vi "Randomize.vi"(11 "Quantity":T1={"Name"="", "Value"=[], "Uncertainty"=[], "Degrees of Freedom"=[], "Correlation"=[], "Randomized uncertainty"=[]}) -> (1 "Canceled?":bool, 3 "Randomized Quantity":T1)   [LabVIEW 2013]
uses:
  qwtblvlib/TD Quantity.ctl
  <vilib>/gmath/statdist.llb/Normal Random.vi
  <vilib>/gmath/statdist.llb/Uniform Random.vi
  <vilib>/gmath/statdist.llb/Triangular Random.vi
  <vilib>/gmath/statdist.llb/Student t Random.vi
  <vilib>/gmath/NI_Gmath.lvlib
  <vilib>/Analysis/NI_AALBase.lvlib
  qwtblvlib/QWTBLVLib.lvlib
panel:
  in  "Repeats":i32=100 min=1 step=1
  out "no dof":bool
  out "msg":string
  in  "reload hist signal":bool
  out "Randomization for quantity:":string
  in  "Maximum - Mean":dbl=1.0 min=0.0
  in  "Mean - Minimum":dbl min=0.0
  in  "Distribution type":T2(ring)
  out "Degrees of freedom":i32=1 min=1
  out "Mean":dbl
  out "Uncertainty":dbl=1.0 min=1e-15
  in  "Seed":i32=-1
  in  "Cancel Button":bool
  in  "OK Button":bool
  out "Example histogram of 1000 samples":T3(graph)
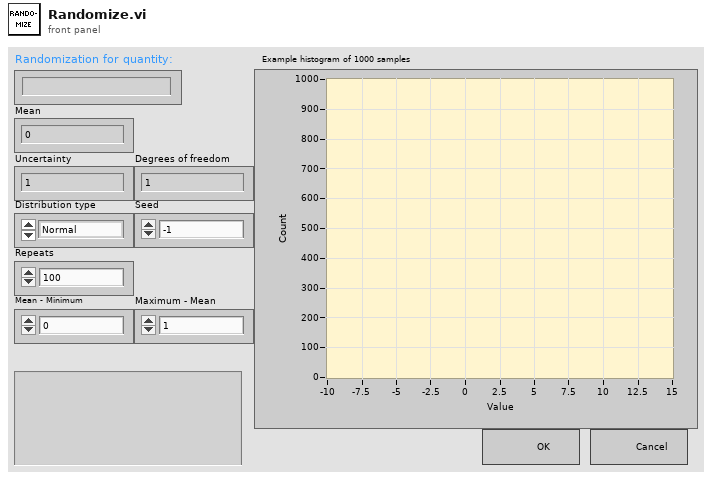
[diagram p1: front panel]
types:
  T1 = typedef "QWTBLVLib.lvlib/TD Quantity.ctl" = cluster{"Name":string, "Value":dbl[][], "Uncertainty":dbl[][], "Degrees of Freedom":dbl[][], "Correlation":dbl[][], "Randomized uncertainty":dbl[][]}
  T2 = enum16{"Normal", "t (Student)", "Triangular", "Uniform"}
  T3 = cluster{"X Values":dbl[], "Histogram: h(x)":i32[]}
  T4 = enum8{"Enabled", "Disabled", "Disabled and Grayed Out"}
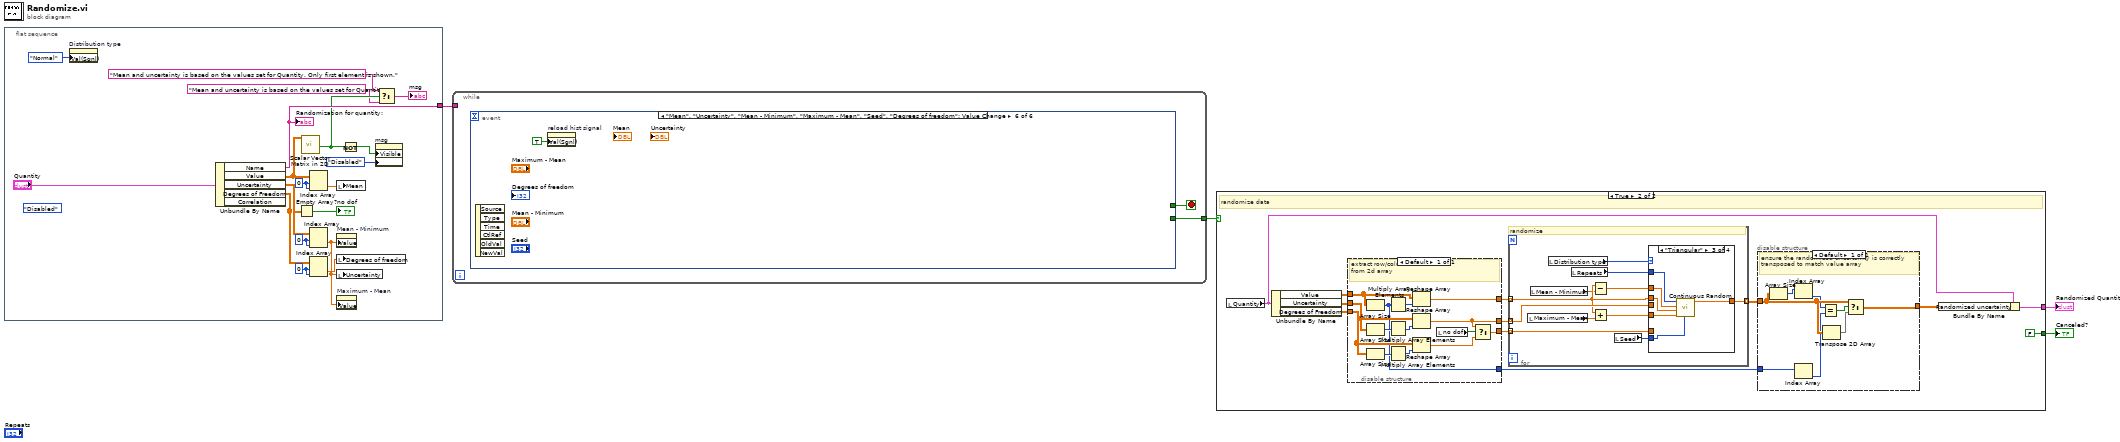
[diagram p0: block diagram]
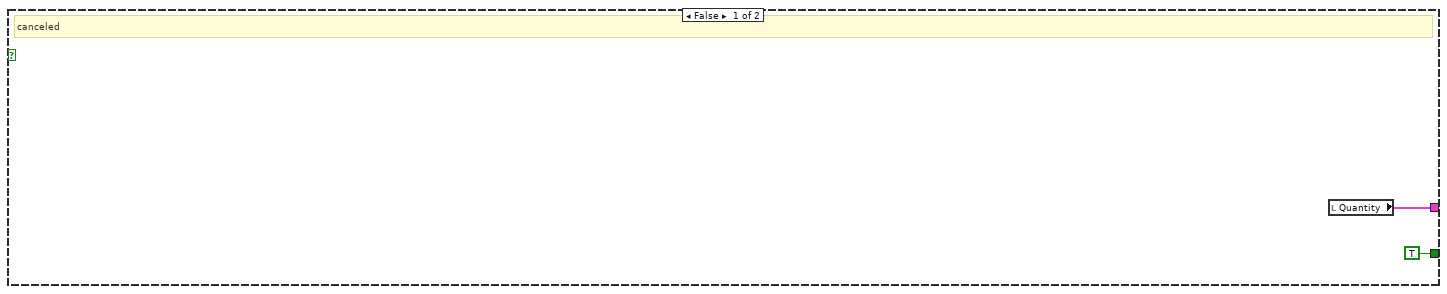
[diagram p2: hidden frame]
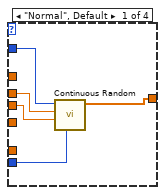
[diagram p3: hidden frame]
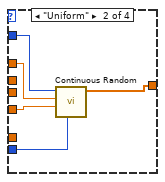
[diagram p4: hidden frame]
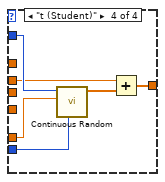
[diagram p5: hidden frame]
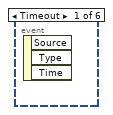
[diagram p6: hidden frame]
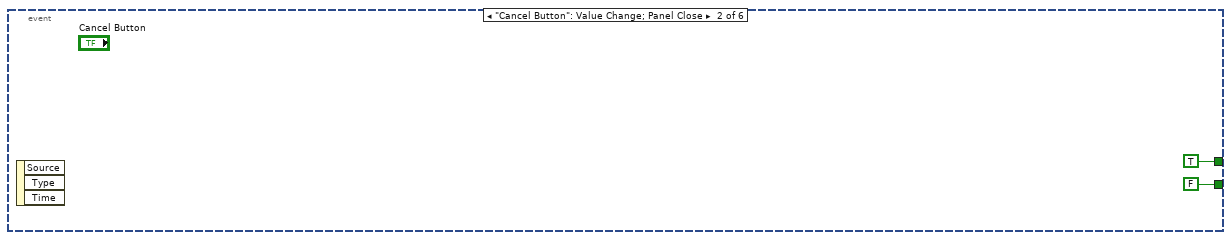
[diagram p7: hidden frame]
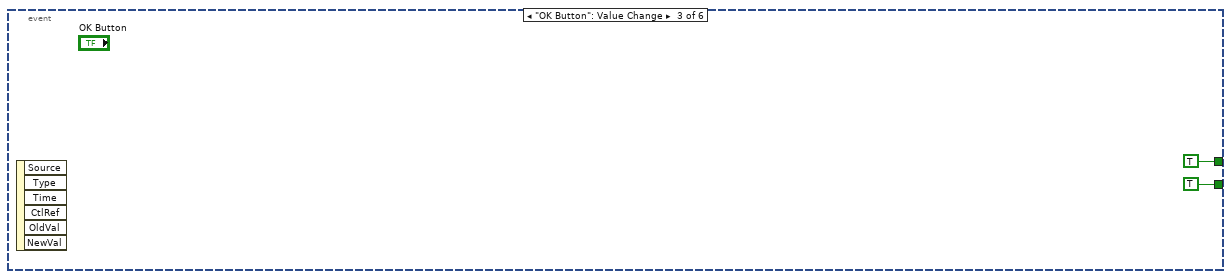
[diagram p8: hidden frame]
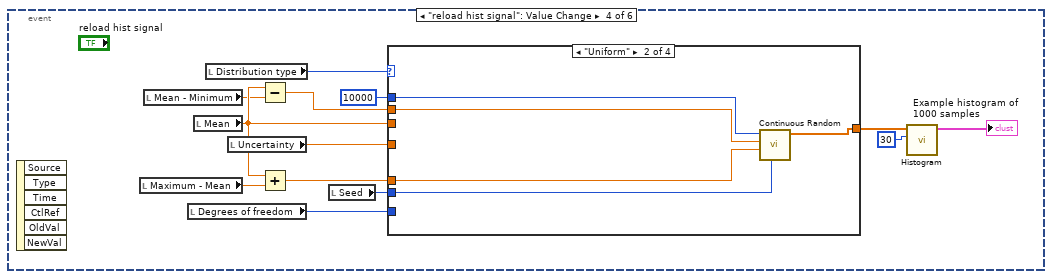
[diagram p9: hidden frame]
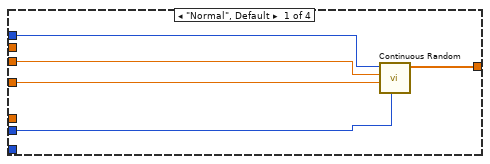
[diagram p10: hidden frame]
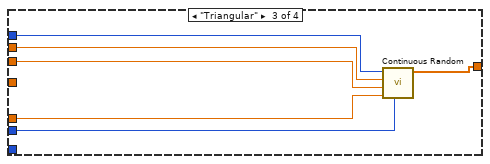
[diagram p11: hidden frame]
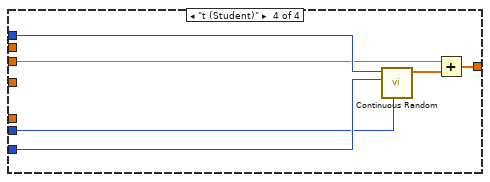
[diagram p12: hidden frame]
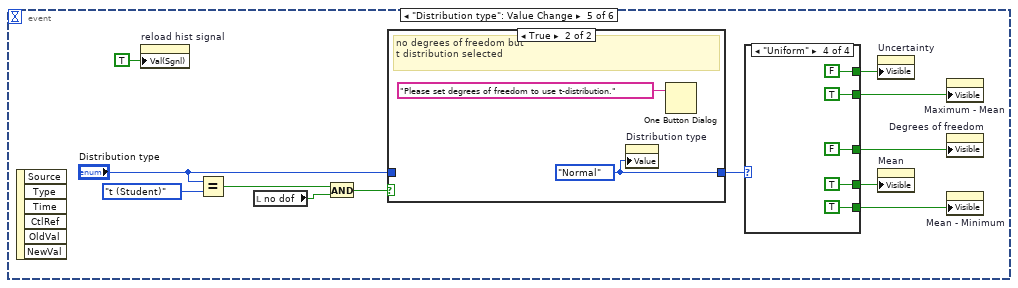
[diagram p13: hidden frame]
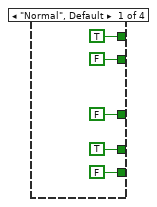
[diagram p15: hidden frame]
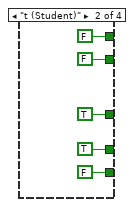
[diagram p16: hidden frame]
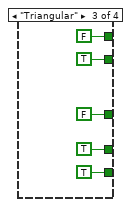
[diagram p17: hidden frame]
diagram:
  n1 = flat-sequence {
    tunnel: [w23] -> w4
    frame #0 {
      w16 = 0 ("index (row)")
      w17 = 0 ("index (row)")
      (unwired) T4."Disabled" ("Disabled")
      w18 = 0 ("index (row)")
      n2 = property on="Distribution type" class="Enum (strict)"("Val(Sgnl)"=T2."Normal" ("Value (Signaling)")) -> ()  [unwired: 2 in, 2 out]
      n3 = Unbundle By Name("Quantity") -> ("Name"=w23:string, "Value"=w11:dbl[][], "Uncertainty"=w21:dbl[][], "Degrees of Freedom"=w19:dbl[][])  [unwired: 1 out]
      "Randomization for quantity:" <- w23
      n4 = Empty Array?(array=w19) -> (empty?=→"no dof":bool)
      n5 = call "Scalar Vector Matrix in 2D.vi"("2D Array"=w11) -> ("Is Vector?"=w10:bool)  [unwired: 4 in, 6 out]
      n6 = Index Array(array=w11, index (row)=w18, index (col)=w18) -> (element=w5:dbl)
      n7 = Index Array(array=w21, index (row)=w17, index (col)=w17) -> (element=w6:dbl)
      n8 = Index Array(array=w19, index (row)=w16, index (col)=w16) -> (element=w15:dbl)
      n9 = local write "Mean"(w5) -> ()
      n10 = property on="Mean - Minimum" class="DigNum (strict)"("Value"=w6) -> ()  [unwired: 2 in, 2 out]
      n11 = local write "Degrees of freedom"(w15) -> ()
      n12 = local write "Uncertainty"(w6) -> ()
      n13 = property on="Maximum - Mean" class="DigNum (strict)"("Value"=w6) -> ()  [unwired: 2 in, 2 out]
      n14 = Not(x=w10) -> (.not. x?=w12:bool)
      n15 = property on="msg" class="Str"("Visible"=w12, "DisabledEnum"=T4."Disabled" ("Disabled")) -> ()  [unwired: 2 in, 2 out]
      n16 = Select(t="Mean and uncertainty is based on the values set for Quantity. Only first element is shown." ("msg scalar"), s=w10, f="Mean and uncertainty is based on the values set for Quantity." ("msg scalar")) -> (s? t:f=→"msg":string)
    }
  }
  n17 = while {
    tunnel: w4 -> [_]
    tunnel: [w24] -> w3
    stop <- w25 stop-if-true
    n18 = event shown="[5] \"Mean\", \"Uncertainty\", \"Mean - Minimum\", \"Maximum - Mean\", \"Seed\", \"Degrees of freedom\": Value Change" {
      selector: _ -> [_ _ _ _ _ _]
      dyn-events: _ -> [_ _ _ _ _ _]
      timeout: _ -> [_ _ _ _ _ _]
      tunnel: [_ TRUE TRUE _ _ _] -> w25
      tunnel: [_ FALSE TRUE _ _ _] -> w24
      event Timeout {
        n19 = event-data() -> ()  [unwired: 1 in, 3 out]
      }
      event "Cancel Button": Value Change; Panel Close {
        n20 = event-data() -> ()  [unwired: 1 in, 3 out]
      }
      event "OK Button": Value Change {
        n21 = event-data() -> ()  [unwired: 1 in, 6 out]
      }
      event "reload hist signal": Value Change {
        n22 = event-data() -> ()  [unwired: 1 in, 6 out]
        n23 = local read "Maximum - Mean"() -> (w34:dbl)
        n24 = local read "Mean - Minimum"() -> (w31:dbl)
        n25 = local read "Degrees of freedom"() -> (w37:i32)
        n26 = local read "Mean"() -> (w32:dbl)
        n27 = local read "Distribution type"() -> (w38:T2)
        n28 = local read "Uncertainty"() -> (w35:dbl)
        n29 = Subtract(x=w32, y=w31) -> (x-y=w30:dbl)
        n30 = Add(x=w32, y=w34) -> (x+y=w33:dbl)
        n31 = local read "Seed"() -> (w36:i32)
        n32 = case shown="\"Uniform\"" w38 {
          tunnel: [w47 w51 w57 w59] -> w42
          tunnel: 10000 ("samples") -> [w46 w52 w56 w64]
          tunnel: w37 -> [_ _ _ w63]
          tunnel: w32 -> [w45 _ w53 w61]
          tunnel: w35 -> [w44 _ _ _]
          tunnel: w36 -> [w43 w50 w58 w62]
          tunnel: w33 -> [_ w49 w54 _]
          tunnel: w30 -> [_ w48 w55 _]
          frame "Normal", Default {
            n33 = call-poly <vilib>:"Continuous Random.vi"("seed"=w43, "std"=w44, "mean"=w45, "samples"=w46) -> ("normal random data"=w47:dbl[])  [unwired: 6 in, 1 out]
          }
          frame "Uniform" {
            n34 = call-poly <vilib>:"Continuous Random.vi"("seed"=w50, "xmax"=w49, "xmin"=w48, "samples"=w52) -> ("uniform random data"=w51:dbl[])  [unwired: 6 in, 1 out]
          }
          frame "Triangular" {
            n35 = call-poly <vilib>:"Continuous Random.vi"("seed"=w58, "xmax"=w54, "xmode"=w53, "xmin"=w55, "samples"=w56) -> ("triangular random data"=w57:dbl[])  [unwired: 5 in, 1 out]
          }
          frame "t (Student)" {
            n36 = call-poly <vilib>:"Continuous Random.vi"("seed"=w62, "k degrees of freedom"=w63, "samples"=w64) -> ("Student t random data"=w60:dbl[])  [unwired: 7 in, 1 out]
            n37 = Add(x=w61, y=w60) -> (x+y=w59:dbl[])
          }
        }
        n38 = call <vilib>:"Histogram.vi"("intervals"=30, "X"=w42) -> ("Histogram Graph"=→"Example histogram of 1000 samples":T3)  [unwired: 6 in, 3 out]
      }
      event "Distribution type": Value Change {
        n39 = event-data() -> ()  [unwired: 1 in, 6 out]
        n40 = property on="reload hist signal" class="Bool (strict)"("Val(Sgnl)"=TRUE ("Value (Signaling)")) -> ()  [unwired: 2 in, 2 out]
        n41 = Equal?(x="Distribution type", y=T2."t (Student)") -> (x = y?=w70:bool)
        n42 = local read "no dof"() -> (w69:bool)
        n43 = And(x=w70, y=w69) -> (x .and. y?=w67:bool)
        n44 = case shown="True" w67 {
          tunnel: [w77 w78] -> w66
          tunnel: "Distribution type" -> [w77 _]
          frame False {
          }
          frame True {
            w78 = T2."Normal" ("y")
            # "no degrees of freedom but\nt distribution selected"
            n45 = property on="Distribution type" class="Enum (strict)"("Value"=w78) -> ()  [unwired: 2 in, 2 out]
            n46 = One Button Dialog(message="Please set degrees of freedom to use t-distribution.") -> ()  [unwired: 1 in, 1 out]
          }
        }
        n47 = case shown="\"Uniform\"" w66 {
          tunnel: [FALSE ("Visible") TRUE ("Visible") FALSE ("Visible") FALSE ("Visible")] -> w76
          tunnel: [FALSE ("Visible") FALSE ("Visible") TRUE ("Visible") TRUE ("Visible")] -> w75
          tunnel: [FALSE ("Visible") FALSE ("Visible") TRUE ("Visible") TRUE ("Visible")] -> w74
          tunnel: [TRUE ("Visible") FALSE ("Visible") FALSE ("Visible") FALSE ("Visible")] -> w73
          tunnel: [TRUE ("Visible") TRUE ("Visible") TRUE ("Visible") TRUE ("Visible")] -> w72
          frame "Normal", Default {
            # "normal"
          }
          frame "t (Student)" {
            # "student"
          }
          frame "Triangular" {
            # "triangular"
          }
          frame "Uniform" {
            # "uniform"
          }
        }
        n48 = property on="Uncertainty" class="DigNum (strict)"("Visible"=w73) -> ()  [unwired: 2 in, 2 out]
        n49 = property on="Mean" class="DigNum (strict)"("Visible"=w72) -> ()  [unwired: 2 in, 2 out]
        n50 = property on="Maximum - Mean" class="DigNum (strict)"("Visible"=w75) -> ()  [unwired: 2 in, 2 out]
        n51 = property on="Degrees of freedom" class="DigNum (strict)"("Visible"=w76) -> ()  [unwired: 2 in, 2 out]
        n52 = property on="Mean - Minimum" class="DigNum (strict)"("Visible"=w74) -> ()  [unwired: 2 in, 2 out]
      }
      event "Mean", "Uncertainty", "Mean - Minimum", "Maximum - Mean", "Seed", "Degrees of freedom": Value Change {
        n53 = event-data() -> ()  [unwired: 1 in, 6 out]
        n54 = property on="reload hist signal" class="Bool (strict)"("Val(Sgnl)"=TRUE ("Value (Signaling)")) -> ()  [unwired: 2 in, 2 out]
      }
    }
  }
  n55 = case shown="True" w3 {
    tunnel: [w102 w112] -> w2
    tunnel: [TRUE ("Canceled?") FALSE ("Canceled?")] -> w1
    frame False {
      # "canceled"
      n56 = local read "Quantity"() -> (w102:T1)
    }
    frame True {
      # "randomize data"
      n57 = local read "Quantity"() -> (w114:T1)
      n58 = Unbundle By Name(w114) -> ("Value"=w111:dbl[][], "Uncertainty"=w107:dbl[][], "Degrees of Freedom"=w106:dbl[][])
      n59 = disable-structure shown="Default" {
        disable-tunnel: w111 -> [w128]
        disable-tunnel: [w126] -> w110
        disable-tunnel: [w115] -> w109
        disable-tunnel: [w117] -> w108
        disable-tunnel: w107 -> [w121]
        disable-tunnel: w106 -> [w120]
        disable-tunnel: [w119] -> w105
        frame Enabled {
          # "extract row/column vectrors\nfrom 2d array"
          n60 = Array Size(array=w128) -> (size(s)=w119:i32[])
          n61 = Array Size(array=w121) -> (size(s)=w124:i32[])
          n62 = Array Size(array=w120) -> (size(s)=w123:i32[])
          n63 = Multiply Array Elements(1:w119) -> (0:w127:i32)
          n64 = Multiply Array Elements(1:w124) -> (0:w125:i32)
          n65 = Multiply Array Elements(1:w123) -> (0:w122:i32)
          n66 = Reshape Array(w128, w127) -> (w126:dbl[])
          n67 = Reshape Array(w121, w125) -> (w117:dbl[])
          n68 = Reshape Array(w120, w122) -> (w116:dbl[])
          n69 = local read "no dof"() -> (w118:bool)
          n70 = Select(t=w117, s=w118, f=w116) -> (s? t:f=w115:dbl[])
        }
      }
      n71 = for {
        tunnel: w110 -> [w141] mode=indexing
        tunnel: w108 -> [w145] mode=indexing
        tunnel: w109 -> [w144] mode=indexing
        tunnel: [w137] -> w103 mode=indexing
        # "randomize"
        n72 = local read "Maximum - Mean"() -> (w143:dbl)
        n73 = local read "Mean - Minimum"() -> (w140:dbl)
        n74 = local read "Distribution type"() -> (w146:T2)
        n75 = local read "Repeats"() -> (w138:i32)
        n76 = Subtract(x=w141, y=w140) -> (x-y=w139:dbl)
        n77 = Add(x=w141, y=w143) -> (x+y=w142:dbl)
        n78 = local read "Seed"() -> (w147:i32)
        n79 = case shown="\"Triangular\"" w146 {
          tunnel: [w152 w156 w162 w164] -> w137
          tunnel: w138 -> [w151 w157 w161 w169]
          tunnel: w144 -> [_ _ _ w168]
          tunnel: w141 -> [w150 _ w158 w166]
          tunnel: w145 -> [w149 _ _ _]
          tunnel: w147 -> [w148 w155 w163 w167]
          tunnel: w142 -> [_ w154 w159 _]
          tunnel: w139 -> [_ w153 w160 _]
          frame "Normal", Default {
            n80 = call-poly <vilib>:"Continuous Random.vi"("seed"=w148, "std"=w149, "mean"=w150, "samples"=w151) -> ("normal random data"=w152:dbl[])  [unwired: 6 in, 1 out]
          }
          frame "Uniform" {
            n81 = call-poly <vilib>:"Continuous Random.vi"("seed"=w155, "xmax"=w154, "xmin"=w153, "samples"=w157) -> ("uniform random data"=w156:dbl[])  [unwired: 6 in, 1 out]
          }
          frame "Triangular" {
            n82 = call-poly <vilib>:"Continuous Random.vi"("seed"=w163, "xmax"=w159, "xmode"=w158, "xmin"=w160, "samples"=w161) -> ("triangular random data"=w162:dbl[])  [unwired: 5 in, 1 out]
          }
          frame "t (Student)" {
            n83 = call-poly <vilib>:"Continuous Random.vi"("seed"=w167, "k degrees of freedom"=w168, "samples"=w169) -> ("Student t random data"=w165:dbl[])  [unwired: 7 in, 1 out]
            n84 = Add(x=w166, y=w165) -> (x+y=w164:dbl[])
          }
        }
      }
      n85 = disable-structure shown="Default" {
        disable-tunnel: w105 -> [w136]
        disable-tunnel: w103 -> [w132]
        disable-tunnel: [w131] -> w104
        frame Enabled {
          # "ensure the randomized uncertainty is correctly\ntransposed to match value array"
          n86 = Array Size(array=w132) -> (size(s)=w135:i32[])
          n87 = Index Array(array=w135) -> (element=w130:i32)  [unwired: 1 in]
          n88 = Index Array(array=w136) -> (element=w129:i32)  [unwired: 1 in]
          n89 = Equal?(x=w130, y=w129) -> (x = y?=w134:bool)
          n90 = Transpose 2D Array(2D array=w132) -> (transposed array=w133:dbl[][])
          n91 = Select(t=w132, s=w134, f=w133) -> (s? t:f=w131:dbl[][])
        }
      }
      n92 = Bundle By Name(cluster=w114, "Randomized uncertainty"=w104) -> (w112:T1)
    }
  }
  "Randomized Quantity" <- w2
  "Canceled?" <- w1
